vi "Configure Output Trigger.vi"(0 "VISA resource name":refnum<visa-resource-name>, 1 "Trigger Location (0: Idle-ARM)":i32(ring) items=["Idle-ARM", "ARM-Trigger", "Trigger-Acquire", "Trigger-Transient"], 2 "Trigger Timing (2: Both)":i32(ring)=2 items=["Before", "After", "Both"], 5 "Channel (0: Channel 1)":i32(ring) items=["Channel 1", "Channel 2"], 7 "Enable Trigger Output (F: Disable)":bool, 9 "Trigger Signal (0: EXT1)":i32(ring) items=["EXT1", "EXT2", "EXT3", "EXT4", "EXT5", "EXT6", "EXT7", "EXT8", "EXT9", "EXT10", "EXT11", "EXT12", "EXT13", "EXT14", "LAN", "INT1", "INT2"], 11 "error in (no error)":errorcluster, 12 "Device Action (2: Both)":i32(ring)=2 items=["Acquire", "Transient", "Both"]) -> (4 "VISA resource name out":refnum<visa-resource-name>, 15 "error out":errorcluster)   [LabVIEW 2020, in "Agilent B2900 Series.lvlib"]
doc: "Configures output triggers for status change between idle-arm, arm-trigger or trigger-action layer. B2900 provides the trigger output function by using the Digital I/O connector on the rear panel"
uses:
  Agilent B2900 Series.lvlib
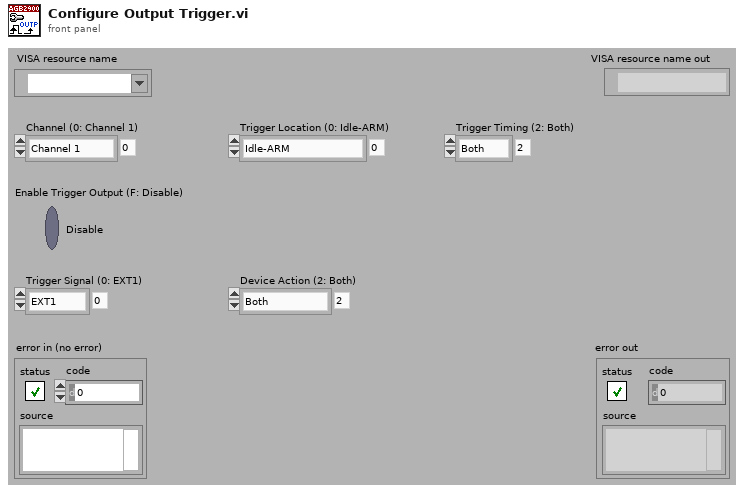
[diagram p1: front panel]
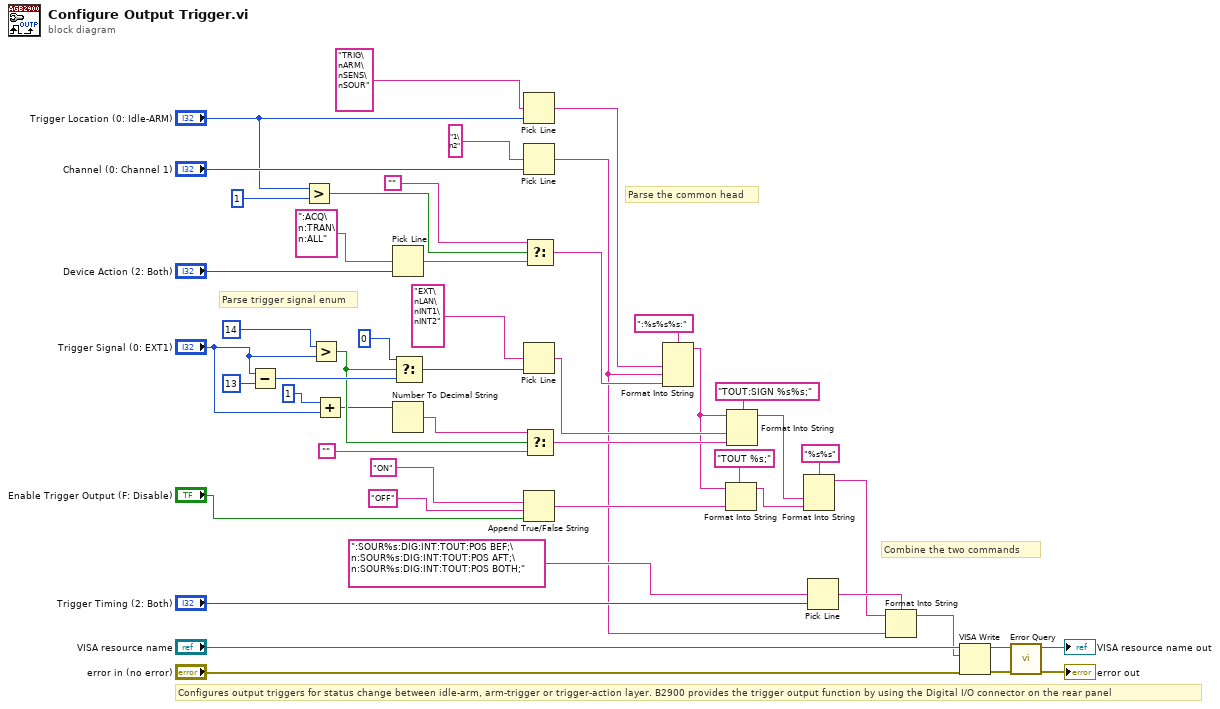
[diagram p0: block diagram]
diagram:
  # "Configures output triggers for status change between idle-arm, arm-trigger or trigger-action layer. B2900 provides the trigger output function by using the Digital I/O connector on the rear panel"
  # "Combine the two commands"
  # "Parse the common head"
  # "Parse trigger signal enum"
  n1 = Subtract(x="Trigger Signal (0: EXT1)", y=13) -> (x-y=w29:i32)
  n2 = Greater?(x="Trigger Location (0: Idle-ARM)", y=1) -> (0:w20:bool)
  n3 = Greater?(x=14 ("y"), y="Trigger Signal (0: EXT1)") -> (0:w26:bool)
  n4 = Add(x=1, y="Trigger Signal (0: EXT1)") -> (x+y=w8:i32)
  n5 = Pick Line(multi-line string=":ACQ\n:TRAN\n:ALL" ("string (\"\")"), line index="Device Action (2: Both)") -> (output string=w19:string)  [unwired: 1 in]
  n6 = Number To Decimal String(number=w8) -> (decimal integer string=w34:string)  [unwired: 1 in]
  n7 = Select(t=0, s=w26, f=w29) -> (s? t:f=w31:i32)
  n8 = Pick Line(multi-line string="TRIG\nARM\nSENS\nSOUR", line index="Trigger Location (0: Idle-ARM)") -> (output string=w24:string)  [unwired: 1 in]
  n9 = Pick Line(multi-line string="1\n2" ("string (\"\")"), line index="Channel (0: Channel 1)") -> (output string=w4:string)  [unwired: 1 in]
  n10 = Pick Line(multi-line string="EXT\nLAN\nINT1\nINT2", line index=w31) -> (output string=w14:string)  [unwired: 1 in]
  n11 = Append True/False String(1:"Enable Trigger Output (F: Disable)", 2:"OFF", 3:"ON") -> (0:w11:string)  [unwired: 1 in]
  n12 = Select(t="", s=w20, f=w19) -> (s? t:f=w17:string)
  n13 = Select(t=w34, s=w26, f="") -> (s? t:f=w15:string)
  n14 = Format Into String(format string=":%s%s%s:" ("string (\"\")"), w24, w4, w17) -> (resulting string=w13:string)  [unwired: 2 in, 1 out]
  n15 = Format Into String(format string="TOUT %s;", initial string=w13, w11) -> (resulting string=w7:string)  [unwired: 1 in, 1 out]
  n16 = Format Into String(format string="TOUT:SIGN %s%s;", initial string=w13, w14, w15) -> (resulting string=w5:string)  [unwired: 1 in, 1 out]
  n17 = Format Into String(format string="%s%s", w5, w7) -> (resulting string=w1:string)  [unwired: 2 in, 1 out]
  n18 = Pick Line(multi-line string=":SOUR%s:DIG:INT:TOUT:POS BEF;\n:SOUR%s:DIG:INT:TOUT:POS AFT;\n:SOUR%s:DIG:INT:TOUT:POS BOTH;", line index="Trigger Timing (2: Both)") -> (output string=w3:string)  [unwired: 1 in]
  n19 = Format Into String(format string=w3, initial string=w1, w4) -> (resulting string=w2:string)  [unwired: 1 in, 1 out]
  n20 = VISA Write(VISA resource name="VISA resource name", write buffer=w2, error in (no error)="error in (no error)") -> (VISA resource name out=w42:refnum<visa-resource-name>, error out=w41:errorcluster)  [unwired: 1 out]
  n21 = call "Error Query.vi"("error in (no error)"=w41, "VISA resource name"=w42) -> ("error out"=→"error out":errorcluster, "VISA resource name out"=→"VISA resource name out":refnum<visa-resource-name>)  [unwired: 6 in, 2 out]
